vi "VisualInspectionCondenser.vi"(8 "error in (no error)":errorcluster, 9 "PN":u16, 10 "SubTestName":string[](array[string])=["Verification of Components Not Installed", "Manufacturing Defects", "DC Input Current Drawn", "12V", "5V", "3.3V", "1.8V", "Reverse Polarity Test - DC Input Current", "Weight Check", "J3.B to Chassis", "J1.16 to Chassis", "J1 Body to Chassis", "J2  Body to Chassis", "J3  Body to Chassis", "J1.17 to J1.18", "Sealing Test", "Mounting Holes Test - Jig Fit"], 11 "TableRef":refnum<vi>) -> (0 "error out":errorcluster, 2 "VisualInspectionResult":bool)   [LabVIEW 2017]
panel:
  in  "7.2.2 2":bool
  in  "6.2.1.1":bool
  in  "6.1.2":bool
  in  "6.1.1":bool
  in  "Cancel Button":bool
  in  "OK Button":bool
  in  "6.2.2.1":bool
  in  "6.2.2.2":bool
  in  "6.2.2.3":bool
  in  "6.2.2.4":bool
  in  "7.1":bool
  in  "7.2.2":bool
  in  "7.2.1":bool
  in  "7.5.1.1":bool
  out "Ring 3":u16(ring)
  in  "Tab Control":T1(tab)
  # "0 - Namer 30 & Warior\n1 - Namer 60\n2 - Condenser"
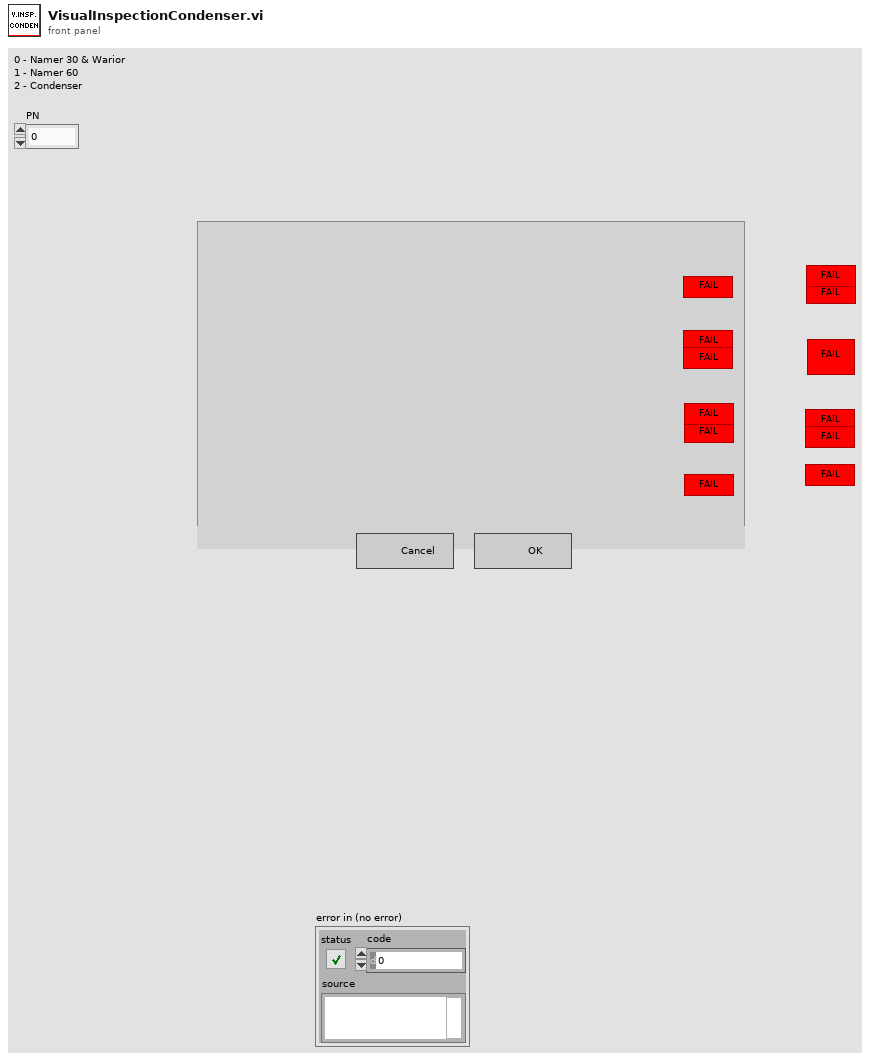
[diagram p1: front panel]
types:
  T1 = enum32{"Namer30,Warrior", "Namer60", "Condenser"}
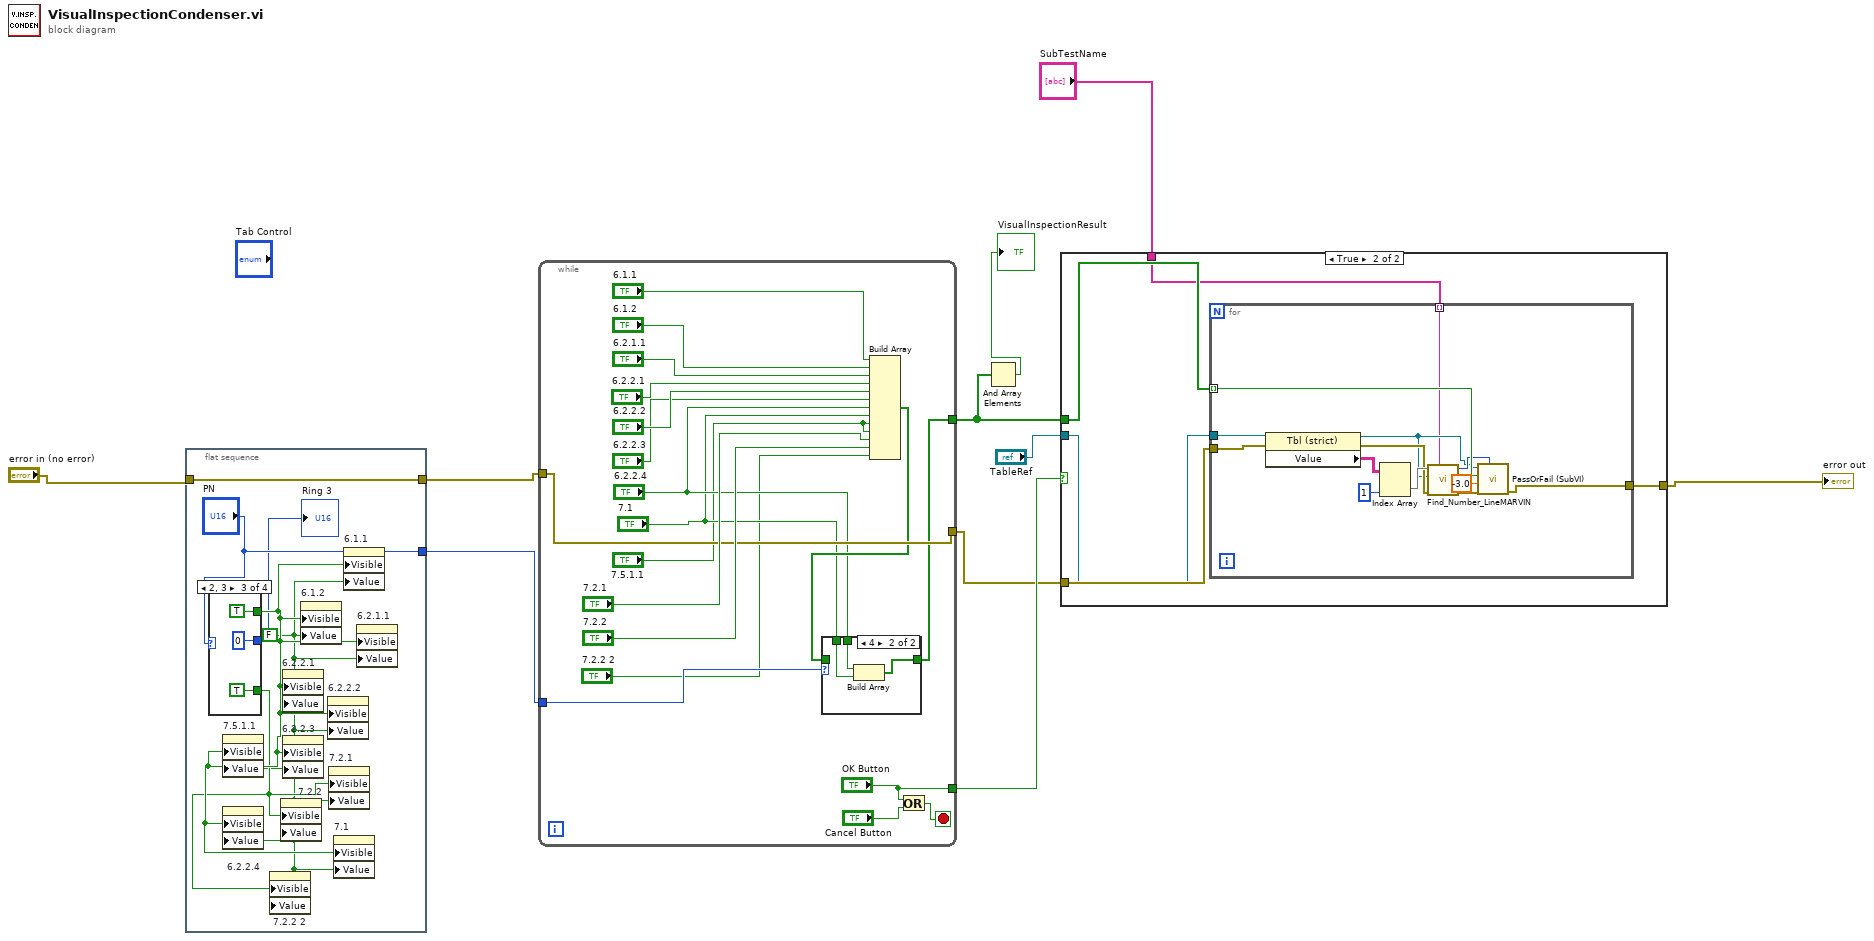
[diagram p0: block diagram]
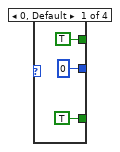
[diagram p2: hidden frame]
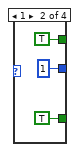
[diagram p3: hidden frame]
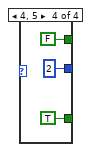
[diagram p4: hidden frame]
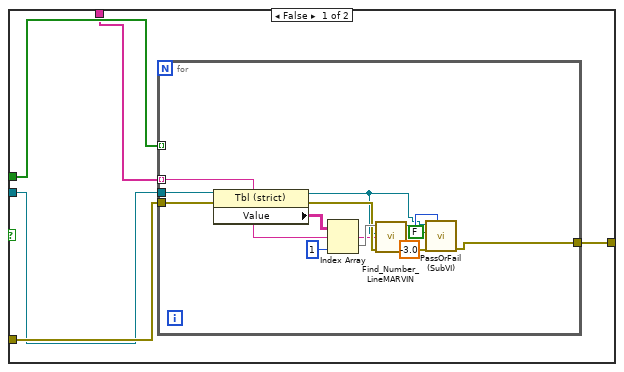
[diagram p5: hidden frame]
diagram:
  n1 = flat-sequence {
    tunnel: "error in (no error)" -> [w16]
    tunnel: [w16] -> w2
    tunnel: ["PN"] -> w1
    frame #0 {
      w12 = FALSE ("6.1.2")
      n2 = case shown="2, 3" "PN" {
        tunnel: [TRUE TRUE TRUE FALSE] -> w15
        tunnel: [TRUE TRUE TRUE TRUE] -> w13
        tunnel: [0 1 0 2] -> w11
        frame 0, Default {
        }
        frame 1 {
        }
        frame 2, 3 {
        }
        frame 4, 5 {
        }
      }
      "Ring 3" <- w11
      n3 = property on="7.5.1.1" class="Bool (strict)"("Visible"=w15, "Value"=w12) -> ()  [unwired: 2 in, 2 out]
      n4 = property on="6.2.2.4" class="Bool (strict)"("Visible"=w15, "Value"=w12) -> ()  [unwired: 2 in, 2 out]
      n5 = property on="7.2.2 2" class="Bool (strict)"("Visible"=w13, "Value"=w12) -> ()  [unwired: 2 in, 2 out]
      n6 = property on="7.2.2" class="Bool (strict)"("Visible"=w13, "Value"=w12) -> ()  [unwired: 2 in, 2 out]
      n7 = property on="6.2.2.1" class="Bool (strict)"("Visible"=w15, "Value"=w12) -> ()  [unwired: 2 in, 2 out]
      n8 = property on="6.2.2.3" class="Bool (strict)"("Visible"=w15, "Value"=w12) -> ()  [unwired: 2 in, 2 out]
      n9 = property on="6.1.2" class="Bool (strict)"("Visible"=w15, "Value"=w12) -> ()  [unwired: 2 in, 2 out]
      n10 = property on="6.2.2.2" class="Bool (strict)"("Visible"=w15, "Value"=w12) -> ()  [unwired: 2 in, 2 out]
      n11 = property on="7.2.1" class="Bool (strict)"("Visible"=w13, "Value"=w12) -> ()  [unwired: 2 in, 2 out]
      n12 = property on="7.1" class="Bool (strict)"("Visible"=w15, "Value"=w12) -> ()  [unwired: 2 in, 2 out]
      n13 = property on="6.1.1" class="Bool (strict)"("Visible"=w15, "Value"=w12) -> ()  [unwired: 2 in, 2 out]
      n14 = property on="6.2.1.1" class="Bool (strict)"("Visible"=w15, "Value"=w12) -> ()  [unwired: 2 in, 2 out]
    }
  }
  n15 = while {
    tunnel: w2 -> [w36]
    tunnel: [w33] -> w5
    tunnel: ["OK Button"] -> w10
    tunnel: [w36] -> w9
    tunnel: w1 -> [w35]
    stop <- w46 stop-if-true
    n16 = Build Array("6.1.1", "6.1.2", "6.2.1.1", "6.2.2.1", "6.2.2.2", "6.2.2.3", "6.2.2.4", "7.1", "7.5.1.1", "7.5.1.1", "7.2.1", "7.2.2", "7.2.2 2") -> (w34:bool[])
    n17 = case shown="4" w35 {
      tunnel: w34 -> [w48 _]
      tunnel: [w48 w49] -> w33
      tunnel: "6.2.2.4" -> [_ w51]
      tunnel: "7.1" -> [_ w50]
      frame 0, Default {
      }
      frame 4 {
        n18 = Build Array(w51, w50) -> (w49:bool[])
      }
    }
    n19 = Or(x="OK Button", y="Cancel Button") -> (x .or. y?=w46:bool)
  }
  n20 = And Array Elements(Boolean array=w5) -> (logical AND=→"VisualInspectionResult":bool)
  n21 = case shown="True" w10 {
    tunnel: w5 -> [w56 w74]
    tunnel: w9 -> [w55 w73]
    tunnel: [w54 w72] -> w6
    tunnel: "TableRef" -> [w53 w71]
    tunnel: "SubTestName" -> [w52 w70]
    frame False {
      n22 = for {
        tunnel: w52 -> [w65] mode=indexing
        tunnel: w56 -> [_] mode=indexing
        tunnel: w55 -> [w62]
        tunnel: [w61] -> w54
        tunnel: w53 -> [w60]
        n23 = property class="Tbl (strict)"(reference=w60, error in=w62) -> (reference out=w57:refnum<vi>, error out=w66:errorcluster, "Value"=w69:string[][])
        n24 = Index Array(array=w69, index (col)=1 ("disabled index (col)")) -> (element=w67:string[])  [unwired: 1 in]
        n25 = call "Find_Number_LineMARVIN.vi"("Test Paragraph"=w65, "error in"=w66, "TableIn"=w57, "Row Headers[]"=w67) -> ("error out"=w64:errorcluster, "Line number"=w63:i32)  [unwired: 1 in, 2 out]
        n26 = call "PassOrFail (SubVI).vi"("index (row)"=w63, "error in (no error)"=w64, "Data in"=-3.0, "Pass?Fail"=FALSE ("Boolean"), "Table in"=w57) -> ("error out"=w61:errorcluster)  [unwired: 5 in, 1 out]
      }
    }
    frame True {
      n27 = for {
        tunnel: w74 -> [w82] mode=indexing
        tunnel: w73 -> [w80]
        tunnel: [w79] -> w72
        tunnel: w71 -> [w78]
        tunnel: w70 -> [w75] mode=indexing
        n28 = property class="Tbl (strict)"(reference=w78, error in=w80) -> (reference out=w76:refnum<vi>, error out=w84:errorcluster, "Value"=w87:string[][])
        n29 = Index Array(array=w87, index (col)=1 ("disabled index (col)")) -> (element=w85:string[])  [unwired: 1 in]
        n30 = call "Find_Number_LineMARVIN.vi"("Test Paragraph"=w75, "error in"=w84, "TableIn"=w76, "Row Headers[]"=w85) -> ("error out"=w83:errorcluster, "Line number"=w81:i32)  [unwired: 1 in, 2 out]
        n31 = call "PassOrFail (SubVI).vi"("index (row)"=w81, "error in (no error)"=w83, "Data in"=-3.0, "Pass?Fail"=w82, "Table in"=w76) -> ("error out"=w79:errorcluster)  [unwired: 5 in, 1 out]
      }
    }
  }
  "error out" <- w6
